vi "sample_ppl_subvi.vi"() -> (3 "Hello World":string)   [LabVIEW 2020, in "sample_ppl.lvlib"]
uses:
  sample_ppl.lvlib
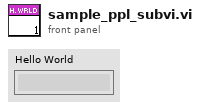
[diagram p1: front panel]
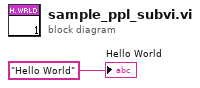
[diagram p0: block diagram]
diagram:
  "Hello World" <- "Hello World" ("Hello World")
